vi "Frequency Drift 3-31.vi"() -> ()   [LabVIEW 2015]
doc: "This VI demonstrates a simple procedure for setting up a spectrum analyzer, running an acquisition, and retrieving and plotting the waveform data.\n\nString indicators Binary WF Data and Sgl Float WF Data are initialized to empty strings. Waveform Graph is initialized to 0 for 100000 locations (just an arbitrary number for demonstration purposes).\n\ntkrsa6100 Initialize.vi opens the VISA Resource Name from the information entered by the user. It also presets the instrument by default to the Spectrum measurement. On completion it passes dup VISA Resource Name and error out to the following drivers.\n\nThe next VI to execute is tkrsa6100 Config Frequency.vi. Numeric control Center Freq (MHz)(50) is passed to the VI to set the center frequency to the default 50MHz value. The Set/Read Freq Setting (Set) is not wired since it defaults to SET, which is what is desired in this case. This is the case for all the configuration VI's in the example.\n\nThe next VI to execute is tkrsa6100 Config Spectrum Settings.vi. Enumerated control Spectrum Settings (CENTER FREQUENCY) is passed a Frequency Span constant and numeric control Freq Span (MHz) (40) to set the span to 40MHz.\n\nNext the reference level is set using tkrsa6100 Config RF Input.vi. Enumerated control Input Setting (REFERENCE LEVEL) is passed a Reference Level constant and numeric control Ref Level (dBm)(0) to set the reference level to 0dBm.\n\nNext the acquisition mode is set to single acquisition using tkrsa6100 Config Acquisition.vi. No parameters are passed since the default setting of this VI sets the acquisition mode to single.\n\nA single acquisition is then performed using tkrsa6100 Run Single Acquisition.vi. This VI sends an INIT command followed by a *OPC? Query. When the acquisition is completed the instrument returns a 1 and the next vi executes.\n\nThe binary waveform data is then retrieved by tkrsa6100 Spectrum Msmt Results.vi. The last acquisition data is retrieved by passing constant GET LAST ACQUISITION RESULT to enumerated input Run Acquisition and/or Get Result (RUN ACQUISITION & GET RESULT). The binary data is converted to a comma separated list of single precision floating point numbers by passing constant YES to enumerated input Convert Resp String (NO). The number of display points (total number of data bytes/4) is passed to a Spectral Display property node to scale the x axis of the graph. The binary data string from output Measurement Response String is copied to string indicator Binary WF Data. The converted binary data from output Converted Sgl Float Response String is copied to string indicator Sgl Float WF Data.\n\nSgl Float WF Data is then converted to an array by function Spreadsheet String to Array using a comma as the data separator. The output array is then passed to waveform graph Spectral Display for viewing.\n\nThe VISA Resource Name is closed using tkrsa6100 Close.vi."
panel:
  in  "Channel Selection":string(combo)
  out "Frequency at end of packet":dbl format="%#_15g"
  out "Drift between measurements":dbl
  out "Frequency at beginning of packet":dbl format="%#_15g"
  in  "VISA Resource Name":refnum<visa-resource-name>
  out "Spectral Display":dbl[](graph)
  out "error out":errorcluster {"code" format="%#.0f"}
  # "RSA6106A/6114A Acquire and Fetch\nSpectral Analysis Display"
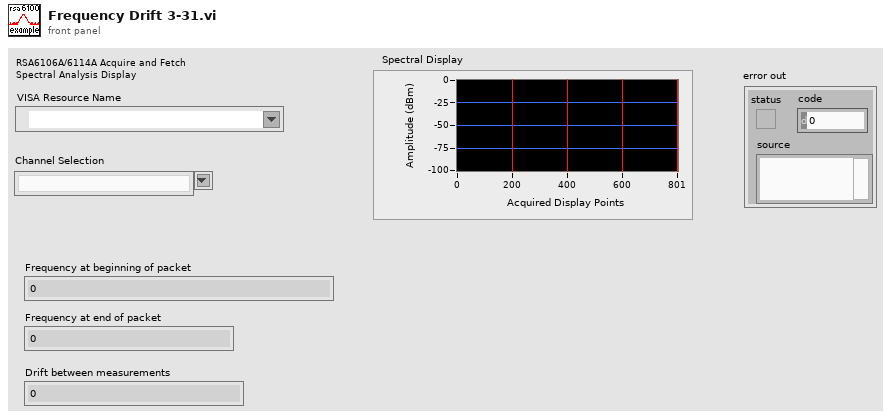
[diagram p1: front panel]
types:
  T1 = enum16{"CENTER FREQUENCY", "FREQUENCY SPAN", "RESOLUTION BW", "MAX REAL TIME SPAN (SET)", "START FREQUENCY", "STOP FREQUENCY", "FREQ STEP SIZE", "AUTO FREQ STEP ON", "AUTO FREQ STEP OFF", "AUTO RES BW ON", "AUTO RES BW OFF", "FFT WINDOW TYPE", "# POINTS", "RBW PROCESS ON", "RBW PROCESS OFF", "GAIN/BW OPTIMIZATION"}
  T2 = enum16{"RUN ACQUISITION  & GET RESULT", "GET LAST ACQUISITION RESULT"}
  T3 = enum16{"ANALYSIS REFERENCE", "ANALYSIS LENGTH", "ACTUAL ANALYSIS LENGTH (READ)", "AUTO ANALYSIS LENGTH ON", "AUTO ANALYSIS LENGTH OFF", "ANALYSIS OFFSET", "AUTO ANALYSIS OFFSET ON", "AUTO ANALYSIS OFFSET OFF", "SPECTRUM LENGTH", "ACTUAL SPECTRUM LENGTH (READ)", "AUTO SPECTRUM LENGTH ON", "AUTO SPECTRUM LENGTH OFF", "SPECTRUM OFFSET", "SPECTRUM TIME MODE", "DITHER MODE", "DITHER HW STATUS (READ)", "AUTO SPECTRUM OFFSETS AND ANALYSIS"}
  T4 = enum16{"TRIGGER SOURCE", "TRIGGER ON", "TRIGGER OFF", "TIME DELAY", "TIME POSITION", "TRIGGER EACH SEGMENT ON", "TRIGGER EACH SEGMENT OFF", "TRIGGER TYPE POWER", "TRIGGER TYPE FREQ MASK", "TRIGGER LEVEL", "TRIGGER SLOPE RISING", "TRIGGER SLOPE FALLING", "TDBW MODE ON", "TDBW MODE OFF", "TDBW", "ACTUAL TDBW (READ)", "CREATE NEW FMT (SET)", "SAVE FMT (SET)", "LOAD FMT (SET)", "FMT VIOLATION LOGIC", "FMT RBW AUTO", "FMT RBW MANUAL", "FMT RBW", "FORCE TRIGGER", "Trigger Position Auto"}
  T5 = enum16{"SPECTRUM ANALYZER", "DPSA", "SPECTROGRAM", "AMPL VS TIME", "FREQ VS TIME", "PHASE VS TIME", "IQ VS TIME", "TIME OVERVIEW"}
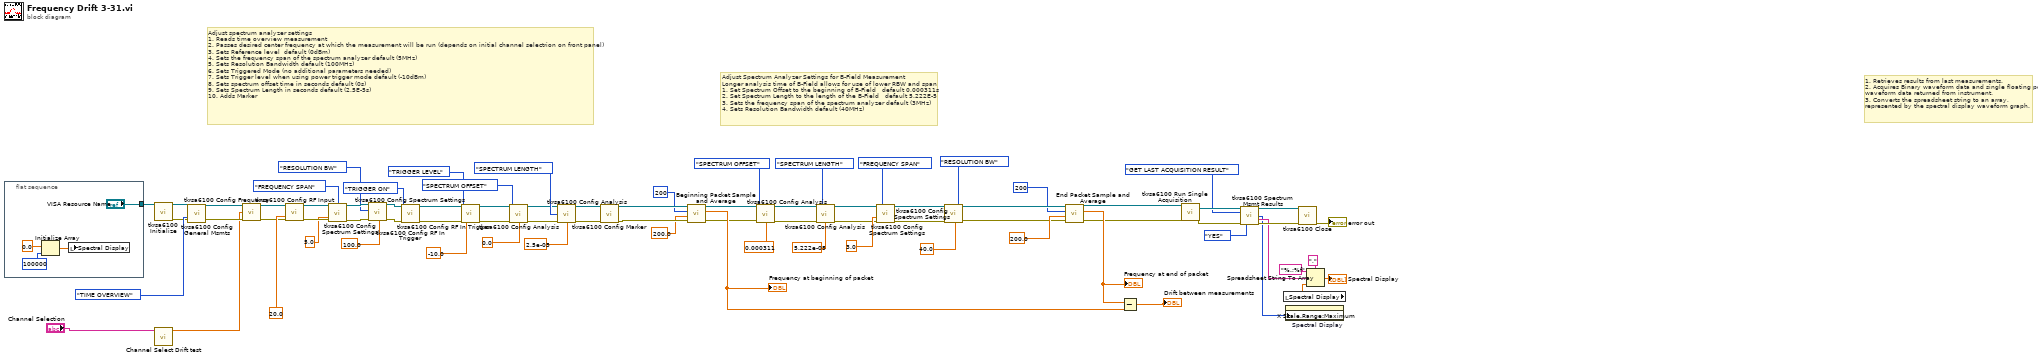
[diagram p0: block diagram]
diagram:
  # "1. Retrieves results from last measurements.\n2. Acquires Binary waveform data and single floating point waveform data returned from instrument.\n3. Converts the spreadsheet string to an array, represented by the spectral display waveform graph."
  # "Adjust Spectrum Analyzer Settings for B-Field Measurement\nLonger analysis time of B-Field allows for use of lower RBW and span\n1. Set Spectrum Offset to the beginning of B-Field   default 0.000311s\n2. Set Spectrum Length to the length of the B-Field   default 5.222E-5\n3. Sets the frequency span of the spectrum analyzer default (3MHz)\n4. Sets Resolution Bandwidth default (40MHz)"
  # "Adjust spectrum analyzer settings\n1. Reads time overview measurement \n2. Passes desired center frequency at which the measurement will be run (depends on initial channel selectrion on front panel)\n3. Sets Reference level  default (0dBm)\n4. Sets the frequency span of the spectrum analyzer default (5MHz)\n5. Sets Resolution Bandwidth default (100MHz)\n6. Sets Triggered Mode (no additional parameters needed)\n7. Sets Trigger level when using power trigger mode default (-10dBm)\n8. Sets spectrum offset time in seconds default (0s)\n9. Sets Spectrum Length in seconds default (2.5E-5s)\n10. Adds Marker"
  n1 = flat-sequence {
    tunnel: ["VISA Resource Name"] -> w69
    frame #0 {
      n2 = Initialize Array(0.0 ("element"), 100000 ("dimension size")) -> (w81:dbl[])
      n3 = local write "Spectral Display"(w81) -> ()
    }
  }
  n4 = call <instrlib>:"tkrsa6100 Initialize.vi"("VISA Resource Name"=w69) -> ("dup VISA Resource Name"=w65:refnum<visa-resource-name>, "error out"=w66:errorcluster)  [unwired: 3 in, 10 out]
  n5 = call "Channel Select Drift test.vi"("Channel Selection"="Channel Selection") -> ("Numeric"=w8:dbl)  [unwired: 10 in]
  n6 = call <instrlib>:"tkrsa6100 Config General Msmts.vi"("VISA Resource Name"=w65, "Measurement\n(SPECTRUM ANALYZER)"=T5."TIME OVERVIEW" ("Measurement\n(SPECTRUM ANALYZER)"), "error in (no error)"=w66) -> ("dup VISA Resource Name"=w50:refnum<visa-resource-name>, "error out"=w49:errorcluster)  [unwired: 10 in, 1 out]
  n7 = call <instrlib>:"tkrsa6100 Config Frequency.vi"("VISA Resource Name"=w50, "Msmt Freq (MHz)\n(1000)"=w8, "error in (no error)"=w49) -> ("dup VISA Resource Name"=w48:refnum<visa-resource-name>, "error out"=w47:errorcluster)  [unwired: 1 in, 10 out]
  n8 = call <instrlib>:"tkrsa6100 Config RF Input.vi"("VISA Resource Name"=w48, "Ref Level (0)"=20.0 ("Ref Level (dBm)(0)"), "error in (no error)"=w47) -> ("dup VISA Resource Name"=w40:refnum<visa-resource-name>, "error out"=w39:errorcluster)  [unwired: 4 in, 7 out]
  n9 = call <instrlib>:"tkrsa6100 Config Spectrum Settings.vi"("VISA Resource Name"=w40, "Spectrum Settings\n (CENTER FREQUENCY)"=T1."FREQUENCY SPAN" ("Spectrum Settings\n (CENTER FREQUENCY)"), "Freq Span\n(MHz)(40)"=5.0 ("Freq Span\n(MHz)(40)"), "error in (no error)"=w39) -> ("dup VISA Resource Name"=w33:refnum<visa-resource-name>, "error out"=w32:errorcluster)  [unwired: 13 in, 1 out]
  n10 = call <instrlib>:"tkrsa6100 Config Spectrum Settings.vi"("VISA Resource Name"=w33, "Spectrum Settings\n (CENTER FREQUENCY)"=T1."RESOLUTION BW" ("Spectrum Settings\n (CENTER FREQUENCY)"), "error in (no error)"=w32, "Res BW (KHz)\n(300)"=100.0 ("Res BW (KHz)\n(300)")) -> ("dup VISA Resource Name"=w31:refnum<visa-resource-name>, "error out"=w30:errorcluster)  [unwired: 13 in, 1 out]
  n11 = call <instrlib>:"tkrsa6100 Config RF In Trigger.vi"("VISA Resource Name"=w31, "Trigger Settings\n(TRIGGER SOURCE)"=T4."TRIGGER ON" ("Trigger Settings\n(TRIGGER SOURCE)"), "error in (no error)"=w30) -> ("dup VISA Resource Name"=w55:refnum<visa-resource-name>, "error out"=w56:errorcluster)  [unwired: 14 in, 1 out]
  n12 = call <instrlib>:"tkrsa6100 Config RF In Trigger.vi"("VISA Resource Name"=w55, "Trigger Settings\n(TRIGGER SOURCE)"=T4."TRIGGER LEVEL" ("Trigger Settings\n(TRIGGER SOURCE)"), "error in (no error)"=w56, "Trig Level\n(dBm)(-10)"=-10.0 ("Trig Level (dBm)")) -> ("dup VISA Resource Name"=w36:refnum<visa-resource-name>, "error out"=w35:errorcluster)  [unwired: 13 in, 1 out]
  n13 = call <instrlib>:"tkrsa6100 Config Analysis.vi"("VISA Resource Name"=w36, "Analysis Setting\n(ANALYSIS REFERENCE)"=T3."SPECTRUM OFFSET" ("Analysis Setting\n(ANALYSIS REFERENCE)"), "error in (no error)"=w35, "Offset Tme (S)(0)"=0.0) -> ("dup VISA Resource Name"=w53:refnum<visa-resource-name>, "error out"=w54:errorcluster)  [unwired: 9 in, 1 out]
  n14 = call <instrlib>:"tkrsa6100 Config Analysis.vi"("VISA Resource Name"=w53, "Length (S)(0.022)"=2.5e-05, "Analysis Setting\n(ANALYSIS REFERENCE)"=T3."SPECTRUM LENGTH" ("Analysis Setting\n(ANALYSIS REFERENCE)"), "error in (no error)"=w54) -> ("dup VISA Resource Name"=w27:refnum<visa-resource-name>, "error out"=w26:errorcluster)  [unwired: 9 in, 1 out]
  n15 = call <instrlib>:"tkrsa6100 Config Marker.vi"("VISA Resource Name"=w27, "error in (no error)"=w26) -> ("dup VISA Resource Name"=w17:refnum<visa-resource-name>, "error out"=w16:errorcluster)  [unwired: 11 in, 1 out]
  n16 = call "Beginning Packet Sample and Average.vi"("error in (no error)"=w16, "y"=200.0, "Numeric in"=200 ("Numeric"), "VISA Refnum in"=w17) -> ("error out"=w5:errorcluster, "Numeric out"=w12:dbl, "VISA Refnum out"=w15:refnum<visa-resource-name>)  [unwired: 5 in]
  "Frequency at beginning of packet" <- w12
  n17 = call <instrlib>:"tkrsa6100 Config Analysis.vi"("VISA Resource Name"=w15, "Analysis Setting\n(ANALYSIS REFERENCE)"=T3."SPECTRUM OFFSET" ("Analysis Setting\n(ANALYSIS REFERENCE)"), "error in (no error)"=w5, "Offset Tme (S)(0)"=0.000311) -> ("dup VISA Resource Name"=w44:refnum<visa-resource-name>, "error out"=w43:errorcluster)  [unwired: 9 in, 1 out]
  n18 = call <instrlib>:"tkrsa6100 Config Analysis.vi"("VISA Resource Name"=w44, "Length (S)(0.022)"=5.222e-05, "Analysis Setting\n(ANALYSIS REFERENCE)"=T3."SPECTRUM LENGTH" ("Analysis Setting\n(ANALYSIS REFERENCE)"), "error in (no error)"=w43) -> ("dup VISA Resource Name"=w19:refnum<visa-resource-name>, "error out"=w18:errorcluster)  [unwired: 9 in, 1 out]
  n19 = call <instrlib>:"tkrsa6100 Config Spectrum Settings.vi"("VISA Resource Name"=w19, "Spectrum Settings\n (CENTER FREQUENCY)"=T1."FREQUENCY SPAN" ("Spectrum Settings\n (CENTER FREQUENCY)"), "Freq Span\n(MHz)(40)"=3.0 ("Freq Span\n(MHz)(40)"), "error in (no error)"=w18) -> ("dup VISA Resource Name"=w23:refnum<visa-resource-name>, "error out"=w22:errorcluster)  [unwired: 13 in, 1 out]
  n20 = call <instrlib>:"tkrsa6100 Config Spectrum Settings.vi"("VISA Resource Name"=w23, "Spectrum Settings\n (CENTER FREQUENCY)"=T1."RESOLUTION BW" ("Spectrum Settings\n (CENTER FREQUENCY)"), "error in (no error)"=w22, "Res BW (KHz)\n(300)"=40.0 ("Res BW (KHz)\n(300)")) -> ("dup VISA Resource Name"=w13:refnum<visa-resource-name>, "error out"=w3:errorcluster)  [unwired: 13 in, 1 out]
  n21 = call "End Packet Sample and Average.vi"("error in (no error)"=w3, "y"=200.0, "dimension size"=200, "VISA Refnum in"=w13) -> ("error out"=w1:errorcluster, "Numeric"=w2:dbl, "VISA Refnum out"=w10:refnum<visa-resource-name>)  [unwired: 5 in]
  "Frequency at end of packet" <- w2
  n22 = Subtract(x=w2, y=w12) -> (x-y=→"Drift between measurements":dbl)
  n23 = call <instrlib>:"tkrsa6100 Run Single Acquisition.vi"("VISA Resource Name"=w10, "error in (no error)"=w1) -> ("dup VISA Resource Name"=w58:refnum<visa-resource-name>, "error out"=w57:errorcluster)  [unwired: 12 out]
  n24 = call <instrlib>:"tkrsa6100 Spectrum Msmt Results.vi"("VISA Resource Name"=w58, "Run Acquisition and/or \nGet Result (RUN ACQUISITION & GET RESULT)"=T2."GET LAST ACQUISITION RESULT" ("Run Acquisition and/or \nGet Result (RUN ACQUISITION & GET RESULT)"), "error in (no error)"=w57, "Convert Resp\nString(NO)"=enum16{"NO", "YES"}."YES" ("Convert Resp\nString(NO)")) -> ("dup VISA Resource Name"=w72:refnum<visa-resource-name>, "# Data Points"=w70:i32, "Converted Sgl Float\nResponse String"=w71:string, "error out"=w74:errorcluster)  [unwired: 7 in, 1 out]
  n25 = local read "Spectral Display"() -> (w78:dbl[])
  n26 = property on="Spectral Display" class="WFGraph (strict)"("X Scale.Range:Maximum"=w70) -> ()  [unwired: 2 in, 2 out]
  n27 = call <instrlib>:"tkrsa6100 Close.vi"("VISA Resource Name"=w72, "error in (no error)"=w74) -> ("error out"=→"error out":errorcluster)  [unwired: 13 out]
  n28 = Spreadsheet String To Array(delimiter (Tab)=",", format string="%.;%f", spreadsheet string=w71, array type (2D Dbl)=w78) -> (array=→"Spectral Display":dbl[])
